vi "Write RX.Data.vi"(8 "error in (no error)":errorcluster, 10 "RX.Data":u8[](array[numeric]) caption="Read Bytes" format="%.0x", 11 "Devices in":refnum<class "Devices.lvclass">) -> (0 "error out":errorcluster, 3 "Devices out":refnum<class "Devices.lvclass">)   [LabVIEW 2020, in "Devices.lvclass"]
uses:
  Devices.lvclass
  Devices.lvclass/Devices.ctl
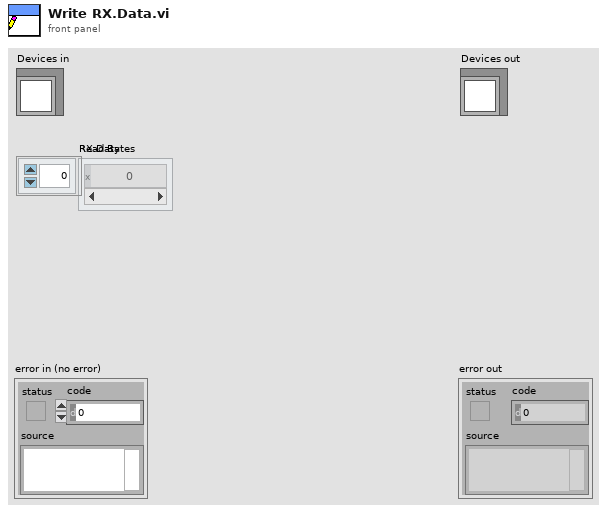
[diagram p1: front panel]
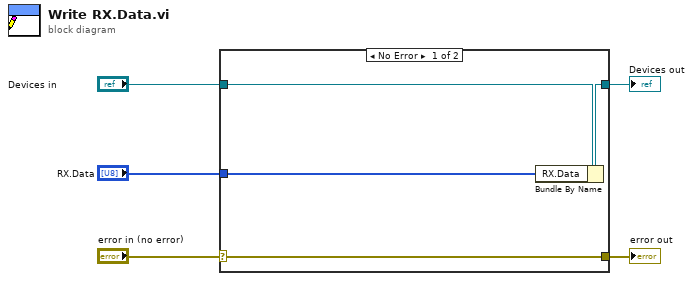
[diagram p0: block diagram]
diagram:
  n1 = case shown="No Error" "error in (no error)" {
    selector: "error in (no error)" -> [w9 w10]
    tunnel: [w9 w10] -> w4
    tunnel: [w7 w11] -> w2
    tunnel: "Devices in" -> [w8 w11]
    tunnel: "RX.Data" -> [w6 _]
    frame No Error {
      n2 = Bundle By Name(cluster=w8, "RX.Data"=w6) -> (w7:refnum<class "Devices.lvclass">)
    }
    frame Error {
    }
  }
  "error out" <- w4
  "Devices out" <- w2
